vi "Logarithmically Spaced Values.vi"(9 "Low Bound":dbl, 10 "High Bound":dbl, 11 "N":i32) -> (3 "Output Array":dbl[](array[numeric]))   [LabVIEW 2019]
panel:
  out "Log-Spaced Values":cluster{i32[], dbl[]}(graph)
  out "Exponents":cluster{i32[], dbl[]}(graph)
  out "Exponents Array":dbl[](array[numeric])
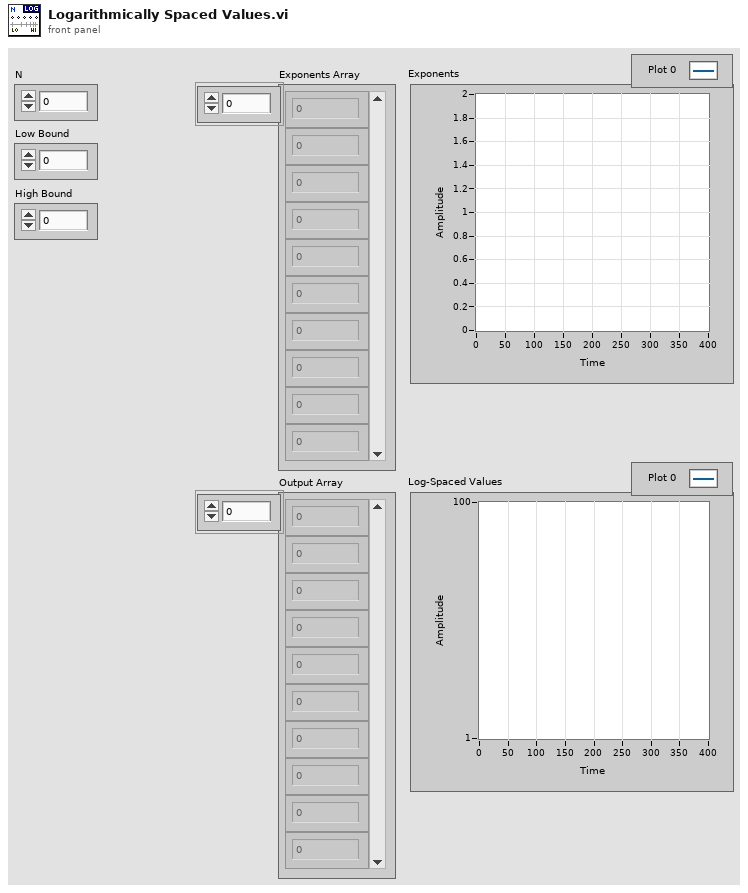
[diagram p1: front panel]
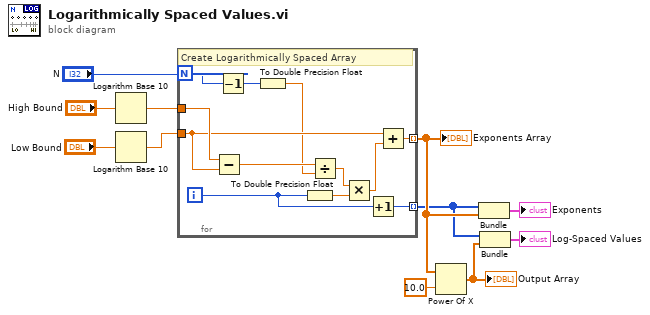
[diagram p0: block diagram]
diagram:
  n1 = Logarithm Base 10(1:"High Bound") -> (0:w4:dbl)
  n2 = Logarithm Base 10(1:"Low Bound") -> (0:w3:dbl)
  n3 = for {
    N: "N" -> [w21]
    tunnel: w3 -> [w18]
    tunnel: w4 -> [w23]
    tunnel: [w17] -> w8 mode=indexing
    tunnel: [w12] -> w7 mode=indexing
    i -> [w14]
    # "Create Logarithmically Spaced Array"
    n4 = Subtract(x=w23, y=w18) -> (x-y=w22:dbl)
    n5 = Decrement(x=w21) -> (x-1=w13:i32)
    n6 = To Double Precision Float(number=w13) -> (double precision float=w16:dbl)
    n7 = To Double Precision Float(number=w14) -> (double precision float=w15:dbl)
    n8 = Divide(x=w22, y=w16) -> (x/y=w20:dbl)
    n9 = Multiply(x=w20, y=w15) -> (x*y=w19:dbl)
    n10 = Increment(x=w14) -> (x+1=w12:i32)
    n11 = Add(x=w18, y=w19) -> (x+y=w17:dbl)
  }
  "Exponents Array" <- w8
  n12 = Power Of X(1:10.0, 2:w8) -> (0:w6:dbl[])
  "Output Array" <- w6
  n13 = Bundle(w7, w8) -> (→"Exponents":cluster{i32[], dbl[]})  [unwired: 1 in]
  n14 = Bundle(w7, w6) -> (→"Log-Spaced Values":cluster{i32[], dbl[]})  [unwired: 1 in]
